vi "Get Possible Connections for Topology.vi"(8 "error in (no error)":errorcluster, 10 "topology":string, 11 "switches json":string) -> (0 "error out":errorcluster, 3 "possible connections":T1[](array[typedef]))   [LabVIEW 2017, in "SLSC Switch System Explorer.lvlib"]
uses:
  SLSC Switch System Explorer.lvlib
  Shared/Routing and Faulting Hardware API/Types/Possible Connections for Endpoint.ctl
  <vilib>/SLSC_Switch/Path Capability.ctl
  <vilib>/SLSC_Switch/Initialize with Topology (Simulate).vi
  <vilib>/SLSC_Switch/SLSC Switch.lvlib
  Shared/Routing and Faulting Hardware API/Routing and Faulting Hardware API.lvlib
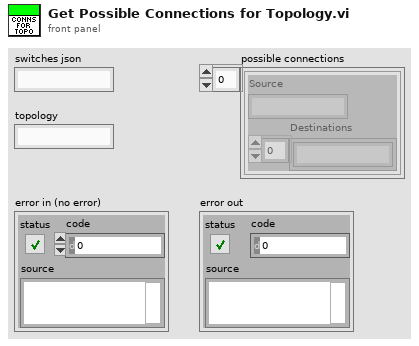
[diagram p1: front panel]
types:
  T1 = typedef "Routing and Faulting Hardware API.lvlib/Possible Connections for Endpoint.ctl" = cluster{"Source":string, "Destinations":string[]}
  T2 = typedef "nislscslSession.ctl" = refnum<k20>
  T3 = typedef "SLSC Switch.lvlib/Path Capability.ctl" = i32
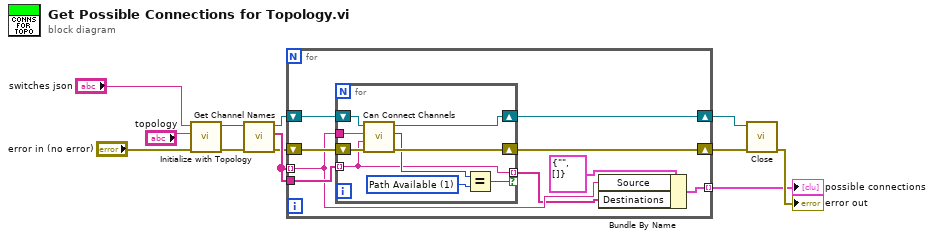
[diagram p0: block diagram]
diagram:
  n1 = call-poly <vilib>:"Initialize with Topology.vi"("error in (no error)"="error in (no error)", "topology"="topology", "switches json"="switches json") -> ("error out"=w4:errorcluster, "session out"=w3:T2)  [unwired: 7 in]
  n2 = call <vilib>:"Get Channel Names.vi"("error in (no error)"=w4, "session in"=w3) -> ("error out"=w6:errorcluster, "channel names"=w7:string[], "session out"=w8:T2)  [unwired: 7 in]
  n3 = for {
    tunnel: [w20] -> w5 mode=indexing
    tunnel: w7 -> [w15] mode=indexing
    tunnel: w7 -> [w19]
    shift-right: [w16] -> w10
    shift-left: w6 -> [w17]
    shift-right: [w13] -> w9
    shift-left: w8 -> [w18]
    n4 = for {
      tunnel: w19 -> [w24] mode=indexing
      shift-right: [w28] -> w16
      shift-left: w17 -> [w29]
      tunnel: w15 -> [w27]
      tunnel: [w24] -> w14 mode=indexing if=w23
      shift-right: [w22] -> w13
      shift-left: w18 -> [w30]
      w25 = T3 1 items=["Path Available"=1, "Path Exists"=2, "Path Unsupported"=3, "Resource in Use"=4, "Source Conflict"=5, "Channel Not Available"=6] ("y")
      n5 = call <vilib>:"Can Connect Channels.vi"("error in (no error)"=w29, "channel 2"=w24, "channel 1"=w27, "session in"=w30) -> ("error out"=w28:errorcluster, "path capability"=w26:T3, "session out"=w22:T2)  [unwired: 5 in]
      n6 = Equal?(x=w26, y=w25) -> (x = y?=w23:bool)
    }
    n7 = Bundle By Name(cluster=T1 {"Source"="", "Destinations"=[]} ("Possible Connections for Endpoint"), "Source"=w15, "Destinations"=w14) -> (w20:T1)
  }
  "possible connections" <- w5
  n8 = call <vilib>:"Close.vi"("error in (no error)"=w10, "session in"=w9) -> ("error out"=→"error out":errorcluster)  [unwired: 9 in]
